vi "StringsToValue(SI).vi"(8 "error in":errorcluster, 10 "input string":string) -> (0 "error out":errorcluster, 2 "Energy/Power(SI)":dbl[](array[numeric]))   [LabVIEW 2012]
uses:
  <vilib>/regexp/Match Regular Expression.xnode
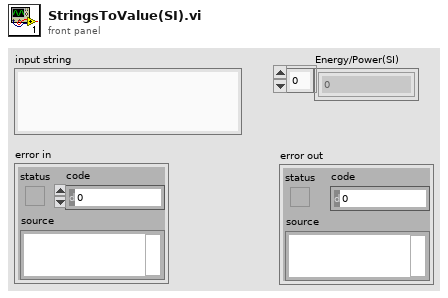
[diagram p1: front panel]
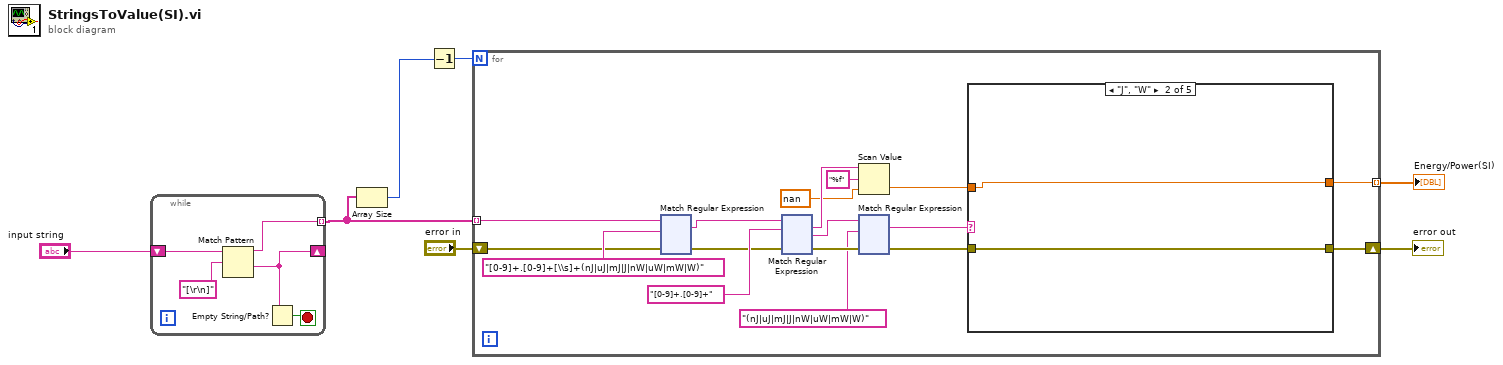
[diagram p0: block diagram]
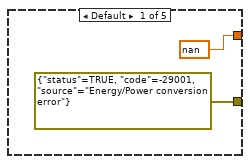
[diagram p2: hidden frame]
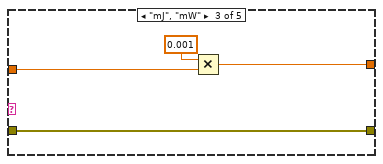
[diagram p3: hidden frame]
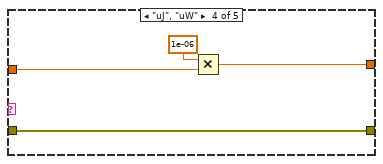
[diagram p4: hidden frame]
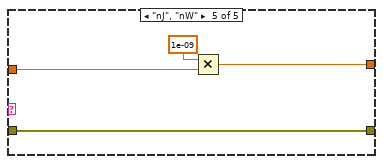
[diagram p5: hidden frame]
diagram:
  n1 = while {
    tunnel: [w10] -> w3 mode=indexing
    shift-right: [w8] -> _
    shift-left: "input string" -> [w12]
    stop <- w9 stop-if-true
    n2 = Match Pattern(string=w12, regular expression="[\r\n]") -> (before substring=w10:string, after substring=w8:string)  [unwired: 1 in, 2 out]
    n3 = Empty String/Path?(string/path=w8) -> (empty?=w9:bool)
  }
  n4 = Array Size(array=w3) -> (size(s)=w2:i32)
  n5 = Decrement(x=w2) -> (x-1=w1:i32)
  n6 = for {
    N: w1 -> [_]
    tunnel: w3 -> [w28] mode=indexing
    shift-right: [w24] -> w5
    shift-left: "error in" -> [w25]
    tunnel: [w23] -> w4 mode=indexing
    n7 = xnode "Match Regular Expression"("input string"=w28, "regular expression"="[0-9]+.[0-9]+[\\s]+(nJ|uJ|mJ|J|nW|uW|mW|W)", "error in"=w25) -> ("whole match"=w15:string, "error out"=w26:errorcluster)  [unwired: 3 in, 3 out]
    n8 = xnode "Match Regular Expression"("input string"=w15, "regular expression"="[0-9]+.[0-9]+", "error in"=w26) -> ("whole match"=w18:string, "after match"=w20:string, "error out"=w22:errorcluster)  [unwired: 3 in, 2 out]
    n9 = Scan Value(string=w18, format string="%f", default (0 dbl)=nan) -> (value=w16:dbl)  [unwired: 1 out]
    n10 = xnode "Match Regular Expression"("input string"=w20, "regular expression"="(nJ|uJ|mJ|J|nW|uW|mW|W)", "error in"=w22) -> ("whole match"=w14:string, "error out"=w21:errorcluster)  [unwired: 3 in, 3 out]
    n11 = case shown="\"J\", \"W\"" w14 {
      tunnel: w21 -> [_ w144 w148 w152 w156]
      tunnel: [errorcluster {"status"=TRUE, "code"=-29001, "source"="Energy/Power conversion error"} ("error out") w144 w148 w152 w156] -> w24
      tunnel: [nan w143 w147 w151 w155] -> w23
      tunnel: w16 -> [_ w143 w145 w149 w153]
      frame Default {
      }
      frame "J", "W" {
      }
      frame "mJ", "mW" {
        n12 = Multiply(x=0.001 ("y"), y=w145) -> (x*y=w147:dbl)
      }
      frame "uJ", "uW" {
        n13 = Multiply(x=1e-06 ("y"), y=w149) -> (x*y=w151:dbl)
      }
      frame "nJ", "nW" {
        n14 = Multiply(x=1e-09 ("y"), y=w153) -> (x*y=w155:dbl)
      }
    }
  }
  "error out" <- w5
  "Energy/Power(SI)" <- w4
